vi "Example1c.vi"() -> ()   [LabVIEW 2011]
uses:
  Interprocess Messenger/QueueMessenger/QueueMessenger.lvclass
  Interprocess Messenger/TextVarientMessage/MSG.lvclass
  Interprocess Messenger/TextVarientMessage/Write (no data).vi
  Interprocess Messenger/Send/Send.lvclass
  Messenging.lvlib
  Interprocess Messenger/SendMultiple/Create Observer.vi
  Interprocess Messenger/SendMultiple/ObserverSet.lvclass
  Parallel Process/Metronome/Metronome.lvclass
  Interprocess Messenger/Send/Send Variant.vi
  Parallel Process/Messsage Logger/Message Logger.lvclass
  Interprocess Messenger/SendOnly/Observer.lvclass
  Parallel Process/ObserverRegister/ObserverRegistry.lvclass
  Interprocess Messenger/TextVarientMessage/Reply (varient).vi
  Interprocess Messenger/TextVarientMessage/Extract Text (static).vi
  Parallel Process/Metronome/Metronome.vi
panel:
  out "Time":string
  # "Stop using the Stop button"
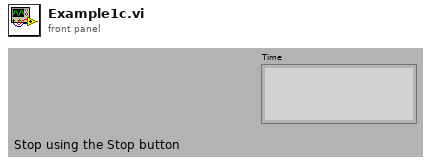
[diagram p1: front panel]
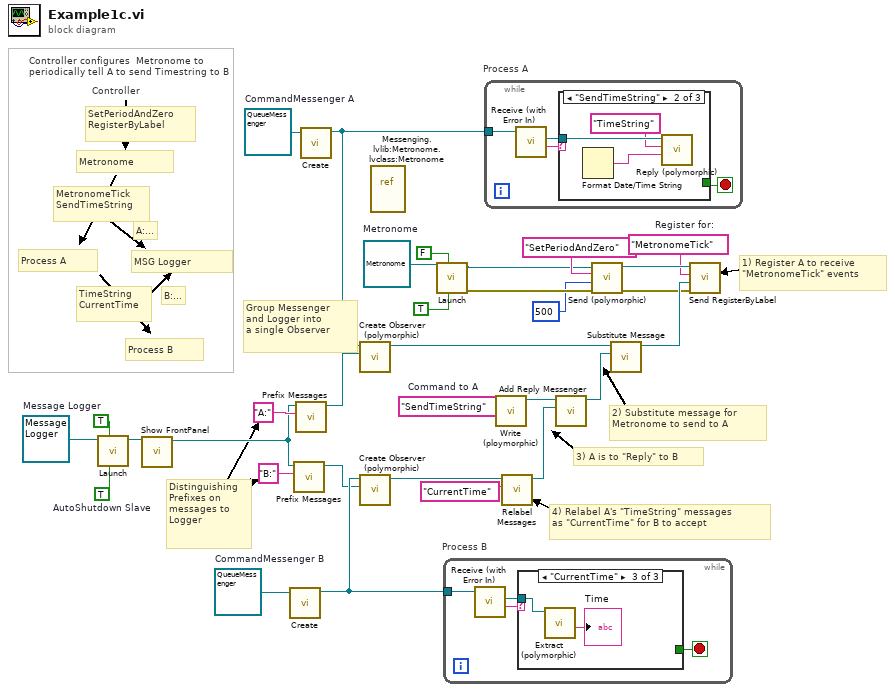
[diagram p0: block diagram]
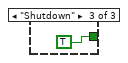
[diagram p3: hidden frame]
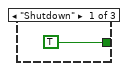
[diagram p4: hidden frame]
diagram:
  w5 = TRUE  # AutoShutdown Slave
  w8 = "MetronomeTick"  # Register for:
  w25 = "SendTimeString"  # Command to A
  w29 = refnum<class "Metronome.lvclass"> refnum  # Metronome
  w3 = refnum<class "Message Logger.lvclass"> refnum  # Message Logger
  w30 = refnum<class "QueueMessenger.lvclass"> refnum  # CommandMessenger A
  w31 = refnum<class "QueueMessenger.lvclass"> refnum  # CommandMessenger B
  # "Group Messenger \nand Logger into \na single Observer"
  # "2) Substitute message for \nMetronome to send to A"
  # "3) A is to \"Reply\" to B"
  # "Distinguishing\nPrefixes on\nmessages to\nLogger"
  # "4) Relabel A's \"TimeString\" messages\nas \"CurrentTime\" for B to accept"
  # "SetPeriodAndZero\nRegisterByLabel"
  # "TimeString \nCurrentTime"
  # "MetronomeTick\nSendTimeString"
  # "Controller"
  # "A:..."
  # "B:..."
  # "1) Register A to receive\n\"MetronomeTick\" events"
  # "MSG Logger"
  # "Controller configures  Metronome to \nperiodically tell A to send Timestring to B"
  # "Process B"
  # "Process A"
  # "Metronome"
  n1 = call-dynamic "Launch.vi"("AutoShutdown Slave (F)"=w5, "Clone if Reentrant (T)"=TRUE, "Parallel Process in"=w3) -> ("Parallel Process out"=w6:refnum<class "Message Logger.lvclass">)  [unwired: 1 in, 7 out]
  n2 = call-dynamic "Show FrontPanel.vi"("Parallel Process in"=w6) -> ("Parallel Process out"=w2:refnum<class "Message Logger.lvclass">)  [unwired: 2 in, 8 out]
  n3 = call-dynamic "Create.vi"("QueueMessenger in"=w31) -> ("QueueMessenger out"=w20:refnum<class "QueueMessenger.lvclass">)  [unwired: 1 in, 9 out]
  n4 = call "Prefix Messages.vi"("Prefix message labels with"="B:" ("Prefix to Add to Label"), "Send IN"=w2) -> ("Observer"=w19:refnum<class "Observer.lvclass">)  [unwired: 1 in, 8 out]
  n5 = call "Prefix Messages.vi"("Prefix message labels with"="A:" ("Prefix to Add to Label"), "Send IN"=w2) -> ("Observer"=w11:refnum<class "Observer.lvclass">)  [unwired: 1 in, 8 out]
  n6 = call-dynamic "Create.vi"("QueueMessenger in"=w30) -> ("QueueMessenger out"=w22:refnum<class "QueueMessenger.lvclass">)  [unwired: 1 in, 9 out]
  n7 = call-poly "Create Observer (polymorphic).vi"("Additional Input"=w11, "Input"=w22) -> ("Observer"=w14:refnum<class "Observer.lvclass">)  [unwired: 7 out]
  n8 = call-poly "Create Observer (polymorphic).vi"("Additional Input"=w19, "Input"=w20) -> ("Observer"=w17:refnum<class "Observer.lvclass">)  [unwired: 7 out]
  n9 = vi-ref "Messenging.lvlib:Metronome.lvclass:Metronome.vi"() -> ()  [unwired: 1 out]
  n10 = call-dynamic "Launch.vi"("AutoShutdown Slave (F)"=TRUE ("Launch as Slave (F)"), "Clone if Reentrant (T)"=FALSE, "Parallel Process in"=w29) -> ("error out"=w24:errorcluster, "Parallel Process out"=w1:refnum<class "Metronome.lvclass">)  [unwired: 1 in, 6 out]
  n11 = while "Process B" {
    tunnel: w20 -> [w35]
    stop <- w32 stop-if-true
    n12 = call-dynamic "Receive (with Error In).vi"("MGR in"=w35) -> ("Label"=w34:string, "Message"=w33:refnum<class "MSG.lvclass">)  [unwired: 2 in, 7 out]
    n13 = case shown="\"CurrentTime\"" w34 {
      tunnel: w33 -> [_ _ w38]
      tunnel: [TRUE _ _] -> w32
      frame "Shutdown" {
      }
      frame Default {
      }
      frame "CurrentTime" {
        n14 = call-poly "Extract (polymorphic).vi"("TextMessage in"=w38) -> ("Text"=→"Time":string)  [unwired: 1 in, 9 out]
      }
    }
  }
  n15 = while "Process A" {
    tunnel: w22 -> [w42]
    stop <- w39 stop-if-true
    n16 = call-dynamic "Receive (with Error In).vi"("MGR in"=w42) -> ("Label"=w41:string, "Message"=w40:refnum<class "MSG.lvclass">)  [unwired: 2 in, 7 out]
    n17 = case shown="\"SendTimeString\"" w41 {
      tunnel: w40 -> [_ w45 _]
      tunnel: [_ _ TRUE] -> w39
      frame "False", Default {
      }
      frame "SendTimeString" {
        n18 = Format Date/Time String() -> (date/time string=w43:string)  [unwired: 3 out]
        n19 = call-poly "Reply (polymorphic).vi"("Varient"=w43, "Reply"="TimeString", "Message to Reply to"=w45) -> ()  [unwired: 1 in, 8 out]
      }
      frame "Shutdown" {
      }
    }
  }
  n20 = call-poly "Write (ploymorphic).vi"("Label"=w25) -> ("Message"=w26:refnum<class "MSG.lvclass">)  [unwired: 1 in, 9 out]
  n21 = call "Relabel Messages.vi"("Relabel messages with"="CurrentTime", "Send IN"=w17) -> ("Observer"=w16:refnum<class "Observer.lvclass">)  [unwired: 9 out]
  n22 = call "Add Reply Messenger.vi"("Reply to..."=w16, "Message"=w26) -> ("Message"=w13:refnum<class "MSG.lvclass">)  [unwired: 1 in, 8 out]
  n23 = call-poly "Send (polymorphic).vi"("error in (no error)"=w24, "Varient"=500, "Label"="SetPeriodAndZero", "MSR Parent in"=w1) -> ("error out"=w7:errorcluster, "MSR Parent out"=w10:refnum<class "Metronome.lvclass">)  [unwired: 6 out]
  n24 = call "Substitute Message.vi"("Substitute Message"=w13, "Send IN"=w14) -> ("Observer"=w9:refnum<class "Observer.lvclass">)  [unwired: 9 out]
  n25 = call "Send RegisterByLabel.vi"("error in (no error)"=w7, "Observer to Register"=w9, "Label"=w8, "MSR Parent in"=w10) -> ()  [unwired: 8 out]
